vi "host-C-1a-1.vi"() -> (0 "K(Indicator)":fxp<+/-,64,32>=1.52587890625e-05, 1 "degree":dbl=-171.37312679332166, 2 "Nominal Freq":fxp<+/-,64,32>=0.494873046875)   [LabVIEW 2012]
uses:
  <vilib>/FPGAPlugInAG/PCI-7831R/niLvFpga_Open_PCI-7831R.vi
  <vilib>/Utility/error.llb/Error Cluster From Error Code.vi
  <vilib>/rvi/errors/niLvFpgaAdjustHostInterfaceError.vi
  <vilib>/FPGAPlugInAG/PCI-7831R/niLvFpga_Abort_PCI-7831R.vi
  <vilib>/FPGAPlugInAG/PCI-7831R/niLvFpga_Close_PCI-7831R.vi
  <vilib>/rvi/interface/nirviOpenFPGA/nirviOpenFPGA.xnode
  SB130-XPS/Documents/FPGA-project-apporach-retraction/FPGA Bitfiles/Apporach-Retract_FPGATarget2_LIAFPGA3a2_iAORjpGRZOA.lvbitx
  LIA_FPGA3a2.vi
  <vilib>/rvi/interface/nirviReadWriteControl/nirviReadWriteControl.xnode
  <vilib>/rvi/interface/nirviMethod/nirviMethod.xnode
  <vilib>/rvi/interface/nirviCloseFPGA/nirviCloseFPGA.xnode
  NiFpgaLv.dll
panel:
  out "Ref":dbl
  out "Sig":dbl
  out "PID Error":fxp<+/-,32,17> format="%.21g"
  out "channelQ":i64
  out "channelI":i64
  in  "Nominal Frequency":dbl=30000.0
  in  "Sampling Frequency Indication":dbl=200000.0
  out "nominal freq. indicator":dbl=0.15
  in  "Tuning Fork Voltage":fxp<+,13,0>=0.010009765625
  in  "Reference Voltage":fxp<+,11,3>=5.0
  in  "stop 3":bool
  in  "Manual Sampling\nFrequency":dbl=200000.0
  out "true f":dbl
  out "VCO Frequency":dbl(graph)
  out "VCO Sine Output":dbl(graph)
  out "VCO Phase":dbl
  in  "Alpha (PID)":dbl=0.0010342 format="%_15g"
  in  "Phase Setpoint":dbl=1.57079632679
  out "Phase":dbl
  out "The Decs":dbl=7.8125e-09
  out "LSB Weight":dbl=0.00030517578125
  in  "K":fxp<+,16,0>=1.52587890625e-05
  in  "nominal freq 2":fxp<+,16,0>=0.154998779296875
  out "x*y":dbl=0.015
  in  "stop 2":bool
  out "3rd stages":i32=1
  out "3rd decimation":i32=977
  out "1st decimation":i32=1
  out "2nd decimation":i32=128
  in  "Time Constant [s]":dbl=2.5 min=0.0 step=0.0001 format="%.2f"
  in  "Filter Rolloff":enum16{"20 dB", "40 dB", "60 dB", "80 dB"}(ring)
  out "Actual Sampling Frequency":dbl=200000.0
  in  "input range of 9205":dbl=10.0
  in  "Sampling Frequency":dbl=200000.0 min=1000.0 max=250000.0
  in  "stop":bool
  out "r":dbl(graph)=7.937638998845702e-07
  out "y":dbl=-1.1906385421752928e-07
  out "x":dbl=-7.84783363342285e-07
  out "f":dbl(graph)=94339.58418667316
  in  "dec2":i16=1
  in  "nominal freq":dbl=30000.0 min=500.0 max=125000.0
  in  "dec1":i16=1000
  in  "stages":i8=1 min=1 max=2
  in  "decimation":i16=1000
  # "Sampling Frequency"
  # "CIC First Decimation"
  # "CIC Second Decimation"
  # "MA Stages"
  # "MA Decimation"
  # "PLL Nominal Frequency"
  # "PLL Frequency Output"
  # "LIA Output"
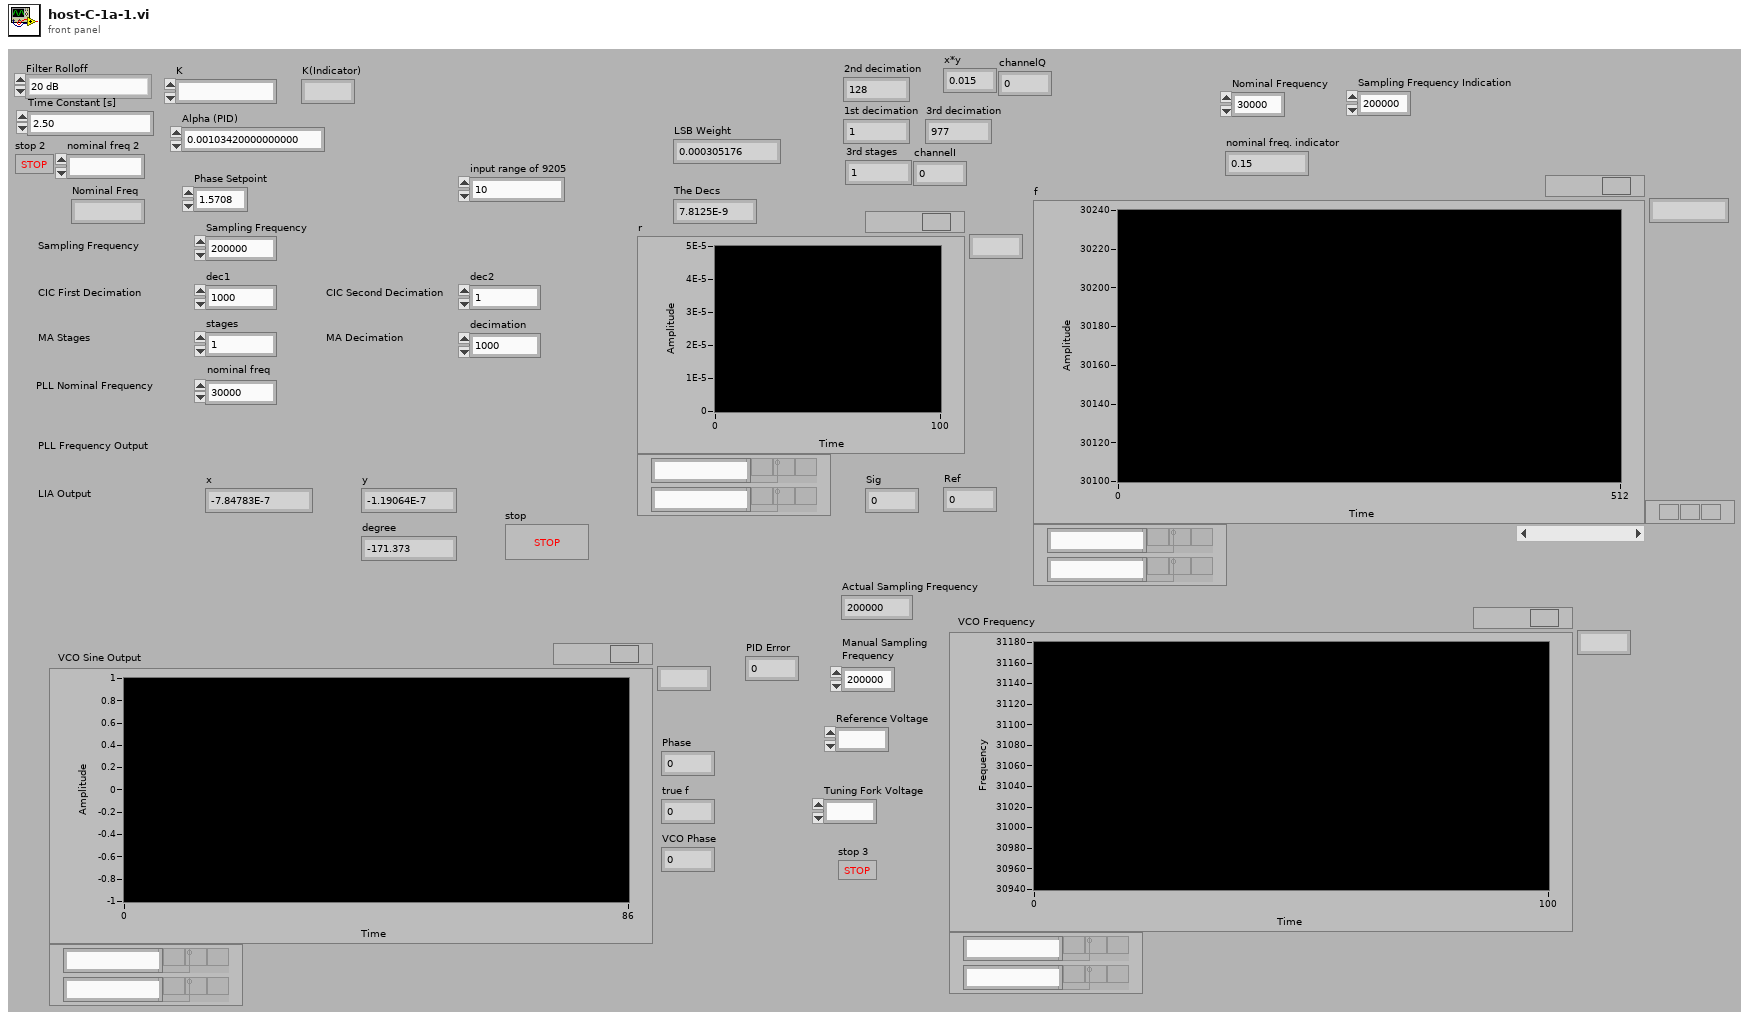
[diagram p1: front panel]
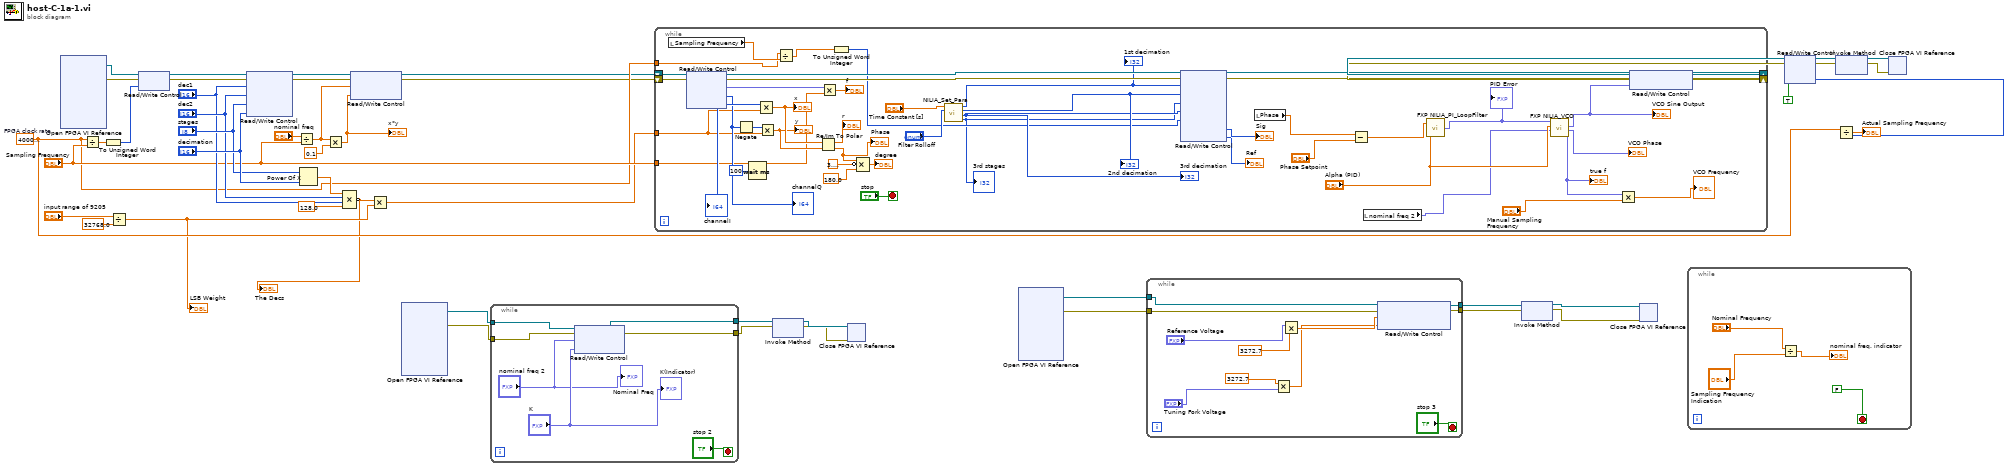
[diagram p0: block diagram]
diagram:
  w19 = 40000000.0  # FPGA clock rate
  n1 = xnode "Open FPGA VI Reference"() -> ("FPGA VI Reference Out"=w25:refnum<k20>, "error out"=w24:errorcluster)  [unwired: 2 in]
  n2 = Divide(x=w19, y="Sampling Frequency") -> (x/y=w31:dbl)
  n3 = To Unsigned Word Integer(number=w31) -> (unsigned 16bit integer=w30:u16)
  n4 = Divide(x="input range of 9205", y=32768.0) -> (x/y=w11:dbl)
  "LSB Weight" <- w11
  n5 = xnode "Read/Write Control"("FPGA VI Reference In"=w25, "error in"=w24, "Period"=w30) -> ("FPGA VI Reference Out"=w33:refnum<k20>, "error out"=w32:errorcluster)
  n6 = xnode "Read/Write Control"("FPGA VI Reference In"=w33, "error in"=w32, "dec1"="dec1", "dec2"="dec2", "stages"="stages", "decimation"="decimation") -> ("FPGA VI Reference Out"=w48:refnum<k20>, "error out"=w47:errorcluster)
  n7 = Divide(x="nominal freq", y="Sampling Frequency") -> (x/y=w27:dbl)
  n8 = Power Of X(1:"decimation", 2:"stages") -> (0:w44:dbl)
  n9 = Multiply(x=w27, y=0.1) -> (x*y=w12:dbl)
  "x*y" <- w12
  n10 = Compound Arithmetic op=MULTIPLY(w44, "dec2", "dec1", 128.0) -> (invert w10:dbl)
  "The Decs" <- w10
  n11 = xnode "Read/Write Control"("FPGA VI Reference In"=w48, "error in"=w47, "nominal freq"=w27, "K"=w12) -> ("FPGA VI Reference Out"=w8:refnum<k20>, "error out"=w7:errorcluster)
  n12 = Multiply(x=w10, y=w11) -> (x*y=w9:dbl)
  n13 = xnode "Open FPGA VI Reference"() -> ("FPGA VI Reference Out"=w18:refnum<k20>, "error out"=w17:errorcluster)  [unwired: 2 in]
  n14 = while {
    tunnel: w18 -> [w54]
    tunnel: w17 -> [w53]
    tunnel: [w52] -> w16
    tunnel: [w51] -> w15
    stop <- "stop 2" stop-if-true
    n15 = xnode "Read/Write Control"("FPGA VI Reference In"=w54, "error in"=w53, "nominal freq"="nominal freq 2", "K"="K") -> ("FPGA VI Reference Out"=w52:refnum<k20>, "error out"=w51:errorcluster)
    "K(Indicator)" <- "K"
    "Nominal Freq" <- "nominal freq 2"
  }
  n16 = while {
    shift-right: [w64] -> w40
    shift-left: w8 -> [w102]
    shift-right: [w63] -> w39
    shift-left: w7 -> [w101]
    tunnel: w9 -> [w98]
    tunnel: "Sampling Frequency" -> [w88]
    tunnel: w19 -> [w77]
    stop <- "stop" stop-if-true
    n17 = local read "Sampling Frequency"() -> (w78:dbl)
    n18 = xnode "Read/Write Control"("FPGA VI Reference In"=w102, "error in"=w101) -> ("FPGA VI Reference Out"=w85:refnum<k20>, "error out"=w84:errorcluster, "f"=w89:fxp<+/-,32,0>, "channelQ"=w99:i64, "channelI"=w100:i64)
    "channelI" <- w100
    "channelQ" <- w99
    n19 = Negate(x=w99) -> (-x=w86:i64)
    n20 = Wait (ms)(milliseconds to wait=u32 100) -> ()  [unwired: 1 out]
    n21 = Multiply(x=w100, y=w98) -> (x*y=w97:dbl)
    "x" <- w97
    n22 = Multiply(x=w86, y=w98) -> (x*y=w96:dbl)
    "y" <- w96
    n23 = Divide(x=w77, y=w78) -> (x/y=w76:dbl)
    n24 = Re/Im To Polar(2:w96, 3:w97) -> (0:w73:dbl, 1:→"r":dbl)
    "Phase" <- w73
    n25 = Multiply(x=w89, y=w88) -> (x*y=→"f":dbl)
    n26 = To Unsigned Word Integer(number=w76) -> (unsigned 16bit integer=w75:u16)
    n27 = Compound Arithmetic op=MULTIPLY(w73, invert 3.141592653589793, 180.0 ("value")) -> (→"degree":dbl)
    n28 = call "NILIA_Set_Para.vi"("rolloff"="Filter Rolloff", "TC [sec]"="Time Constant [s]") -> ("3rd stages"=w74:i32, "3rd decimation"=w79:i32, "2nd decimation"=w80:i32, "1st decimation"=w81:i32)  [unwired: 5 in, 1 out]
    "2nd decimation" <- w80
    "1st decimation" <- w81
    "3rd decimation" <- w79
    "3rd stages" <- w74
    n29 = xnode "Read/Write Control"("FPGA VI Reference In"=w85, "error in"=w84, "dec1"=w81, "dec2"=w80, "stages"=w74, "decimation"=w79, "Period"=w75) -> ("FPGA VI Reference Out"=w66:refnum<k20>, "error out"=w65:errorcluster, "sig"=→"Sig":i16, "ref"=→"Ref":i16)
    n30 = local read "Phase"() -> (w72:dbl)
    n31 = Subtract(x=w72, y="Phase Setpoint") -> (x-y=w71:dbl)
    n32 = local read "nominal freq 2"() -> (w58:fxp<+,16,0>)
    n33 = call "FXP NILIA_PI_LoopFilter.vi"("alpha [U16.-2]"="Alpha (PID)", "x [I16.2]"=w71) -> ("x+y [I32.17]"=w69:fxp<+/-,32,17>)  [unwired: 1 in]
    "PID Error" <- w69
    n34 = call "FXP NILIA_VCO.vi"("nominal freq [U16.0]"=w58, "Kv [U16.0]"="Alpha (PID)", "v [I32.17]"=w69) -> ("f"=w61:fxp<+/-,32,0>, "z [I32.1]"=→"VCO Phase":fxp<+/-,32,1>, "sin(z) [I16.2]"=w62:fxp<+/-,16,2>)  [unwired: 5 in, 1 out]
    "VCO Sine Output" <- w62
    "true f" <- w61
    n35 = Multiply(x=w61, y="Manual Sampling\nFrequency") -> (x*y=→"VCO Frequency":dbl)
    n36 = xnode "Read/Write Control"("FPGA VI Reference In"=w66, "error in"=w65, "VCO Sinz Output"=w62) -> ("FPGA VI Reference Out"=w64:refnum<k20>, "error out"=w63:errorcluster)
  }
  n37 = xnode "Invoke Method"("FPGA VI Reference In"=w16, "error in"=w15) -> ("FPGA VI Reference Out"=w14:refnum<k20>, "error out"=w13:errorcluster)
  n38 = xnode "Close FPGA VI Reference"("FPGA VI Reference In"=w14, "error in"=w13) -> ()  [unwired: 1 out]
  n39 = xnode "Open FPGA VI Reference"() -> ("FPGA VI Reference Out"=w6:refnum<k20>, "error out"=w5:errorcluster)  [unwired: 2 in]
  n40 = while {
    tunnel: w6 -> [w112]
    tunnel: w5 -> [w111]
    tunnel: [w110] -> w2
    tunnel: [w109] -> w1
    stop <- "stop 3" stop-if-true
    n41 = Multiply(x=3272.7, y="Tuning Fork Voltage") -> (x*y=w103:dbl)
    n42 = Multiply(x="Reference Voltage", y=3272.7) -> (x*y=w108:dbl)
    n43 = xnode "Read/Write Control"("FPGA VI Reference In"=w112, "error in"=w111, "Reference Voltage"=w108, "Tuning Fork Voltage"=w103) -> ("FPGA VI Reference Out"=w110:refnum<k20>, "error out"=w109:errorcluster)
  }
  n44 = xnode "Invoke Method"("FPGA VI Reference In"=w2, "error in"=w1) -> ("FPGA VI Reference Out"=w4:refnum<k20>, "error out"=w3:errorcluster)
  n45 = xnode "Close FPGA VI Reference"("FPGA VI Reference In"=w4, "error in"=w3) -> ()  [unwired: 1 out]
  n46 = while {
    stop <- FALSE ("Nominal Frequency") stop-if-true
    n47 = Divide(x="Nominal Frequency", y="Sampling Frequency Indication") -> (x/y=→"nominal freq. indicator":dbl)
  }
  n48 = xnode "Read/Write Control"("FPGA VI Reference In"=w40, "error in"=w39, "stop"=TRUE) -> ("FPGA VI Reference Out"=w37:refnum<k20>, "error out"=w36:errorcluster, "ticks"=w21:u16)
  n49 = xnode "Invoke Method"("FPGA VI Reference In"=w37, "error in"=w36) -> ("FPGA VI Reference Out"=w35:refnum<k20>, "error out"=w34:errorcluster)
  n50 = Divide(x=w19, y=w21) -> (x/y=→"Actual Sampling Frequency":dbl)
  n51 = xnode "Close FPGA VI Reference"("FPGA VI Reference In"=w35, "error in"=w34) -> ()  [unwired: 1 out]
